vi "DrawImage.vi"(8 "Color Table":T1(ring), 10 "Image In":T2) -> (3 "new picture":picture)   [LabVIEW 2019]
uses:
  <vilib>/picture/picture.llb/imagedata.ctl
panel:
  out "Image out":T2
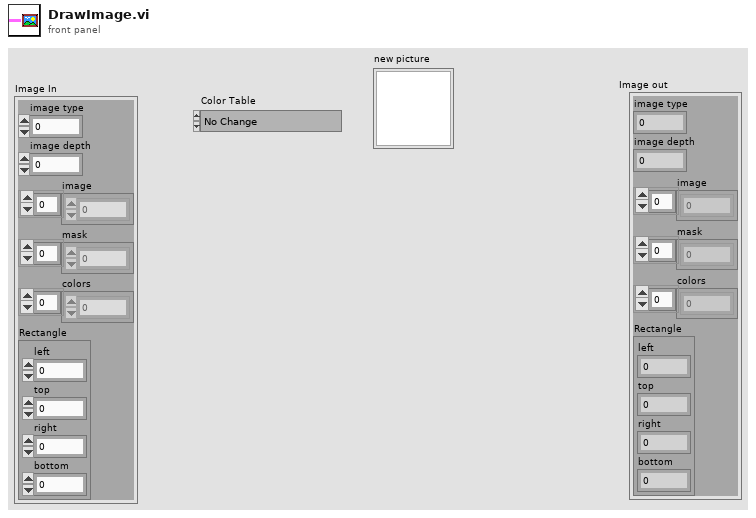
[diagram p1: front panel]
types:
  T1 = enum16{"No Change", "Apricot", "Carnation", "Ether", "Greyscale", "Greyscale-banded", "Hot Metal", "Lava Waves", "Mac", "Morning Glory", "Rainbow", "Rainbow-banded", "Rainbow-inverted", "Rainbow-striped", "Saturn", "Seismic", "Space"}
  T2 = typedef "imagedata.ctl" = cluster{"image type":i32, "image depth":i32, "image":u8[], "mask":u8[], "colors":u32[], "Rectangle":cluster{"left":i16, "top":i16, "right":i16, "bottom":i16}}
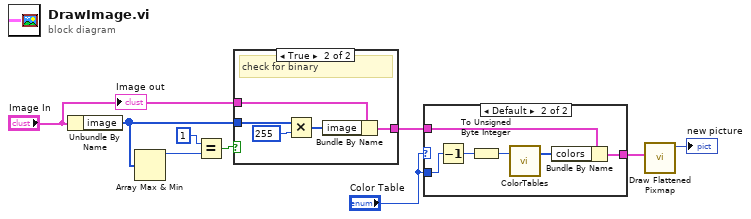
[diagram p0: block diagram]
diagram:
  n1 = Unbundle By Name("Image In") -> ("image"=w4:u8[])
  n2 = Array Max & Min(array=w4) -> (max value=w6:u8)  [unwired: 3 out]
  n3 = Equal?(x=u8 1, y=w6) -> (x = y?=w1:bool)
  n4 = case shown="True" w1 {
    tunnel: w4 -> [_ w15]
    tunnel: "Image In" -> [w10 w12]
    tunnel: [w10 w11] -> w2
    frame False {
    }
    frame True {
      # "check for binary"
      n5 = Multiply(x=w15, y=u8 255 ("x")) -> (x*y=w13:u8[])
      n6 = Bundle By Name(cluster=w12, "image"=w13) -> (w11:T2)
    }
  }
  n7 = case shown="Default" "Color Table" {
    tunnel: w2 -> [w16 w22]
    tunnel: [w16 w20] -> w8
    tunnel: "Color Table" -> [_ w19]
    frame "No Change" {
    }
    frame Default {
      n8 = Decrement(x=w19) -> (x-1=w18:T1)
      n9 = To Unsigned Byte Integer(number=w18) -> (unsigned 8bit integer=w17:u8)
      n10 = call "ColorTables.vi"("Color Table"=w17) -> ("Color Table Out"=w21:u32[])  [unwired: 2 in]
      n11 = Bundle By Name(cluster=w22, "colors"=w21) -> (w20:T2)
    }
  }
  n12 = call <vilib>:"Draw Flattened Pixmap.vi"("image data"=w8) -> ("new picture"=→"new picture":picture)  [unwired: 8 in]
  "Image out" <- "Image In"
